vi "Init Server PS.vi"(8 "error in":errorcluster, 11 "Cfg Handle":T1) -> (0 "error out":errorcluster, 1 "Ozone Out":refnum<k21>, 2 "Filter Out Task":refnum<k21>, 3 "PS Switch Out":refnum<k21>)   [LabVIEW 2015]
uses:
  <userlib>/_Session Fwk/Typedefs/Session Handle.ctl
  <userlib>/_Session Fwk/Session - Root.lvclass
  Controls/Flags.ctl
  Reusable/Session APIs/File Access/Config Data/Config Data.lvclass
  <vilib>/DAQmx/write.llb/DAQmx Write (Digital 1D Bool NChan 1Samp 1Line).vi
  <vilib>/Utility/config.llb/Read Key (Boolean).vi
  <vilib>/DAQmx/miscellaneous.llb/DAQmx Fill In Error Info.vi
  <vilib>/Utility/config.llb/Read Key (I32).vi
  <vilib>/Utility/config.llb/NI_LVConfig.lvlib
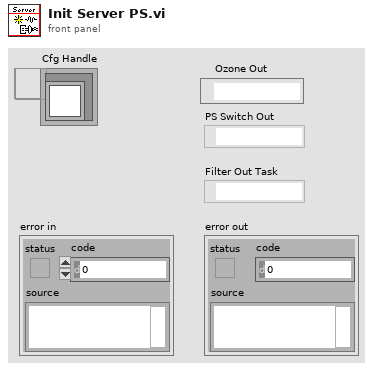
[diagram p1: front panel]
types:
  T1 = typedef "Session - Root.lvclass/Session Handle.ctl" = refnum<data-value>
  T2 = typedef "Flags.ctl" = enum8{"Autospeaker", "Link cycles", "Autofilter", "O3 Cal", "Filter Position"}
  T3 = typedef "NI_LVConfig.lvlib/Config Data RefNum.ctl" = refnum<k1>
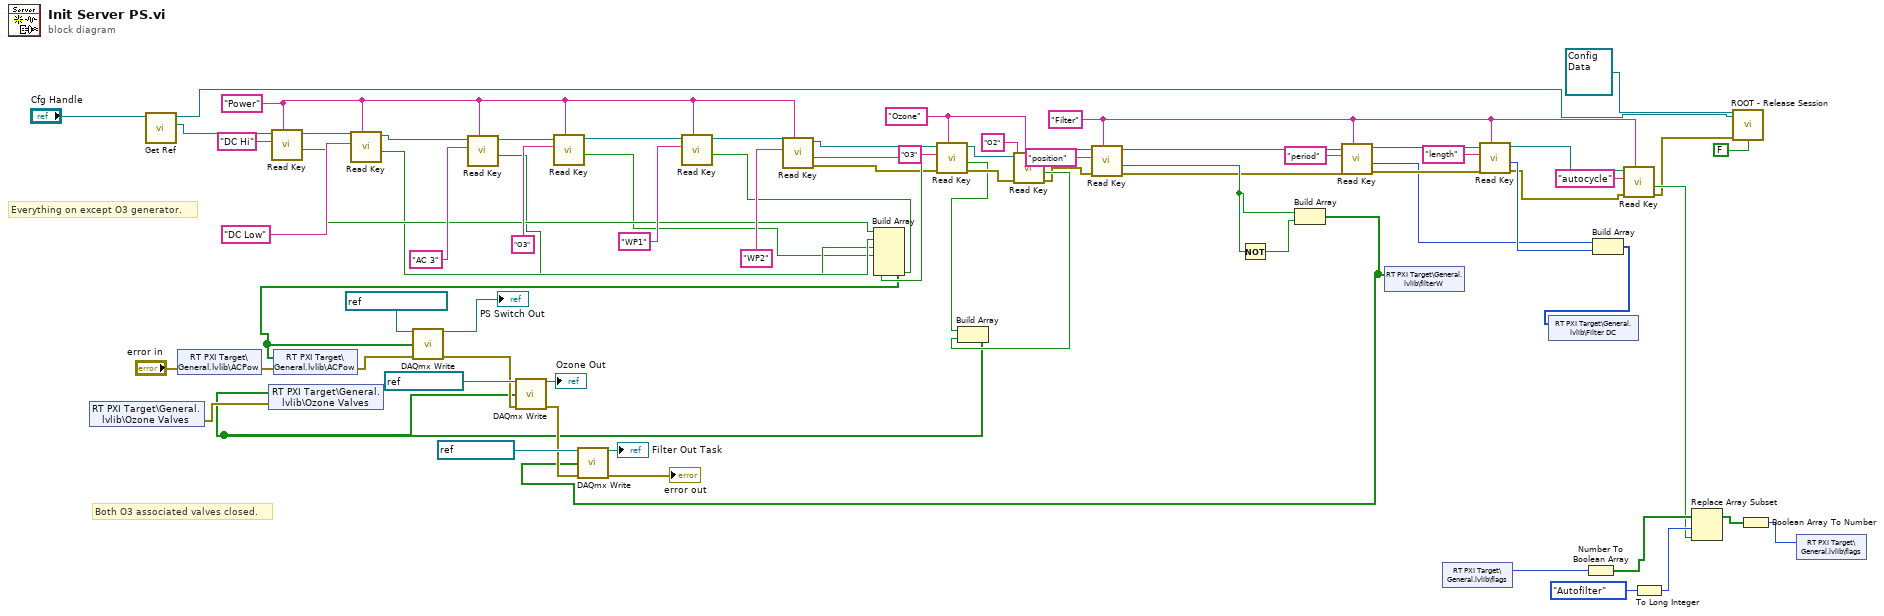
[diagram p0: block diagram]
diagram:
  w13 = "Filter" ("section")
  w34 = "Ozone" ("section")
  w55 = "Power" ("section")
  # "Everything on except O3 generator."
  # "Both O3 associated valves closed."
  n1 = shared-variable "RT PXI Target\\General.lvlib\\Ozone Valves"() -> (error out=w67:errorcluster)  [unwired: 1 in, 1 out]
  n2 = call "Get Ref.vi"("Session Handle In"="Cfg Handle") -> ("Ref"=w60:T3, "Session Handle Out"=w2:T1)  [unwired: 8 in, 1 out]
  n3 = shared-variable "RT PXI Target\\General.lvlib\\ACPow"(error in="error in") -> (error out=w69:errorcluster)  [unwired: 1 out]
  n4 = call-poly <vilib>:"Read Key.vi"("section"=w55, "key"="DC Hi", "refnum"=w60) -> ("value"=w47:bool, "refnum out"=w59:T3)  [unwired: 5 in, 2 out]
  n5 = call-poly <vilib>:"Read Key.vi"("section"=w55, "key"="DC Low", "refnum"=w59) -> ("value"=w46:bool, "refnum out"=w58:T3)  [unwired: 5 in, 2 out]
  n6 = call-poly <vilib>:"Read Key.vi"("section"=w55, "key"="AC 3", "refnum"=w58) -> ("value"=w45:bool, "refnum out"=w57:T3)  [unwired: 5 in, 2 out]
  n7 = call-poly <vilib>:"Read Key.vi"("section"=w55, "key"="O3", "refnum"=w57) -> ("value"=w44:bool, "refnum out"=w56:T3)  [unwired: 5 in, 2 out]
  n8 = call-poly <vilib>:"Read Key.vi"("section"=w55, "key"="WP1", "refnum"=w56) -> ("value"=w43:bool, "refnum out"=w54:T3)  [unwired: 5 in, 2 out]
  n9 = call-poly <vilib>:"Read Key.vi"("section"=w55, "key"="WP2", "refnum"=w54) -> ("error out"=w39:errorcluster, "value"=w42:bool, "refnum out"=w40:T3)  [unwired: 5 in, 1 out]
  n10 = Build Array(w47, w46, w45, w44, w43, w42) -> (w41:bool[])
  n11 = shared-variable "RT PXI Target\\General.lvlib\\ACPow"(w41, error in=w69) -> (error out=w68:errorcluster)
  n12 = call-poly <vilib>:"DAQmx Write.vi"("task/channels in"=refnum<k21> "PS Switch Out" ("DAQmx Task Name"), "data"=w41, "error in"=w68) -> ("task out"=→"PS Switch Out":refnum<k21>, "error out"=w65:errorcluster)  [unwired: 10 in, 1 out]
  n13 = call-poly <vilib>:"Read Key.vi"("section"=w34, "error in (no error)"=w39, "key"="O3", "refnum"=w40) -> ("error out"=w37:errorcluster, "value"=w32:bool, "refnum out"=w38:T3)  [unwired: 4 in, 1 out]
  n14 = call-poly <vilib>:"Read Key.vi"("section"=w34, "error in (no error)"=w37, "key"="O2", "refnum"=w38) -> ("error out"=w29:errorcluster, "value"=w33:bool, "refnum out"=w30:T3)  [unwired: 4 in, 1 out]
  n15 = Build Array(w32, w33) -> (w31:bool[])
  n16 = shared-variable "RT PXI Target\\General.lvlib\\Ozone Valves"(w31, error in=w67) -> ()  [unwired: 1 out]
  n17 = call-poly <vilib>:"DAQmx Write.vi"("task/channels in"=refnum<k21> "O3 Valves", "data"=w31, "error in"=w65) -> ("task out"=→"Ozone Out":refnum<k21>, "error out"=w63:errorcluster)  [unwired: 10 in, 1 out]
  n18 = call-poly <vilib>:"Read Key.vi"("section"=w13, "error in (no error)"=w29, "key"="position", "refnum"=w30) -> ("error out"=w24:errorcluster, "value"=w27:bool, "refnum out"=w25:T3)  [unwired: 4 in, 1 out]
  n19 = Not(x=w27) -> (.not. x?=w28:bool)
  n20 = Build Array(w27, w28) -> (w16:bool[])
  n21 = call-poly <vilib>:"DAQmx Write.vi"("task/channels in"=refnum<k21> "Filter Out" ("DAQmx Task Name"), "data"=w16, "error in"=w63) -> ("task out"=→"Filter Out Task":refnum<k21>, "error out"=→"error out":errorcluster)  [unwired: 10 in, 1 out]
  n22 = call-poly <vilib>:"Read Key.vi"("section"=w13, "error in (no error)"=w24, "key"="period", "refnum"=w25) -> ("error out"=w22:errorcluster, "value"=w18:i32, "refnum out"=w23:T3)  [unwired: 4 in, 1 out]
  n23 = shared-variable "RT PXI Target\\General.lvlib\\filterW"(w16) -> ()  [unwired: 1 in, 1 out]
  n24 = shared-variable "RT PXI Target\\General.lvlib\\flags"() -> (w11:u8)  [unwired: 1 in, 1 out]
  n25 = call-poly <vilib>:"Read Key.vi"("section"=w13, "error in (no error)"=w22, "key"="length", "refnum"=w23) -> ("error out"=w14:errorcluster, "value"=w19:i32, "refnum out"=w15:T3)  [unwired: 4 in, 1 out]
  n26 = Number To Boolean Array(number=w11) -> (Boolean array=w9:bool[])
  n27 = Build Array(w18, w19) -> (w17:i32[])
  n28 = shared-variable "RT PXI Target\\General.lvlib\\Filter DC"(w17) -> ()  [unwired: 1 in, 1 out]
  n29 = call-poly <vilib>:"Read Key.vi"("section"=w13, "error in (no error)"=w14, "key"="autocycle", "refnum"=w15) -> ("error out"=w4:errorcluster, "value"=w7:bool)  [unwired: 4 in, 2 out]
  n30 = To Long Integer(number=Flags."Autofilter") -> (32bit integer=w8:i32)
  n31 = Replace Array Subset(array=w9, new element=w7, index=w8) -> (w6:bool[])
  n32 = call <userlib>:"ROOT - Release Session.vi"("OBJ - Session in"=refnum<class "Config Data.lvclass"> refnum ("Config Data"), "Session Handle in"=w2, "error in (no error)"=w4, "force destroy? (F)"=FALSE) -> ()  [unwired: 10 in, 2 out]
  n33 = Boolean Array To Number(Boolean array=w6) -> (number=w5:u32)
  n34 = shared-variable "RT PXI Target\\General.lvlib\\flags"(w5) -> ()  [unwired: 1 in, 1 out]
